vi "PCO_UserInterfaceSettings.vi"() -> (0 "PCO_UserInterfaceSettings":T2, 1 "PCO_UserInterfaceSettings_Raw":T1, 2 "Length":u16, 3 "Raw_Length":u16)   [LabVIEW 2020, in "SDK.lvlib" / "Structures.lvlib"]
doc: "Use this template to build a VI to use as a subVI."
uses:
  Structures.lvlib
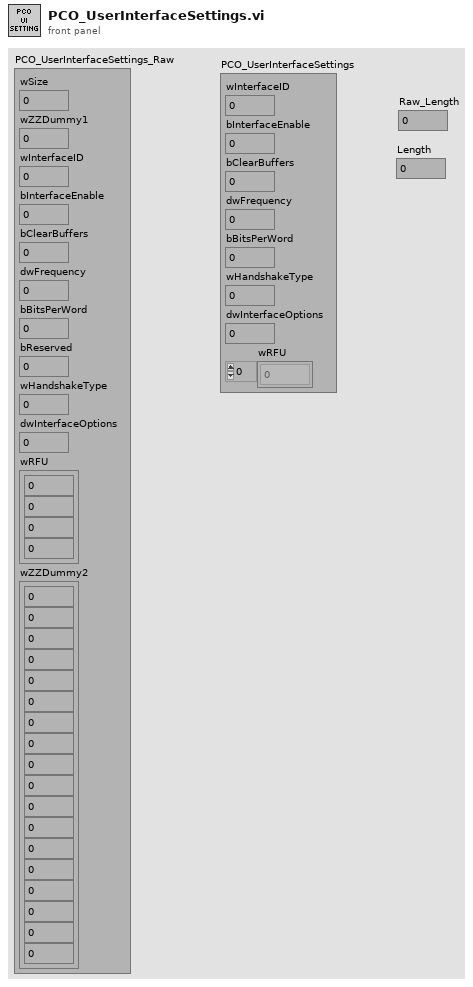
[diagram p1: front panel]
types:
  T1 = cluster{"wSize":u16, "wZZDummy1":u16, "wInterfaceID":u16, "bInterfaceEnable":u8, "bClearBuffers":u8, "dwFrequency":u32, "bBitsPerWord":u8, "bReserved":u8, "wHandshakeType":u16, "dwInterfaceOptions":u32, "wRFU":cluster{u16, u16, u16, u16}, "wZZDummy2":cluster{u16, u16, u16, u16, u16, u16, u16, u16, u16, u16, u16, u16, u16, u16, u16, u16, u16, u16}}
  T2 = cluster{"wInterfaceID":u16, "bInterfaceEnable":u8, "bClearBuffers":u8, "dwFrequency":u32, "bBitsPerWord":u8, "wHandshakeType":u16, "dwInterfaceOptions":u32, "wRFU":u16[]}
  T3 = cluster{u16, u16, u16, u16, u16, u16, u16, u16, u16, u16, u16, u16, u16, u16, u16, u16, u16, u16}
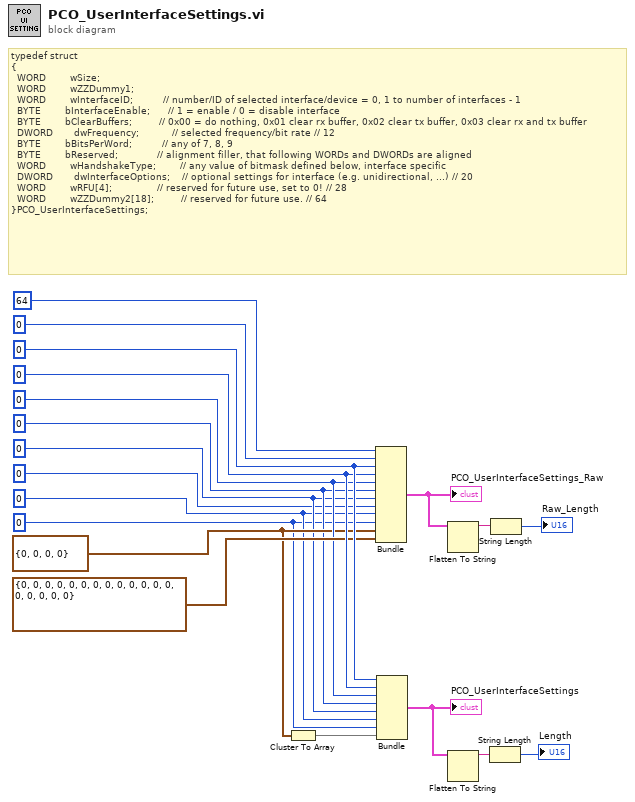
[diagram p0: block diagram]
diagram:
  w7 = cluster{u16, u16, u16, u16} {0, 0, 0, 0} ("wRFU")
  w2 = u32 0 ("dwInterfaceOptions")
  w3 = u16 0 ("wHandshakeType")
  w5 = u8 0 ("bBitsPerWord")
  w6 = u32 0 ("dwFrequency")
  w9 = u8 0 ("bClearBuffers")
  w12 = u8 0 ("bInterfaceEnable")
  w13 = u16 0 ("wInterfaceID")
  # "typedef struct\n{\n  WORD        wSize;\n  WORD        wZZDummy1;\n  WORD        wInterfaceID;          // number/ID of selected interface/device = 0, 1 to number of interfaces - 1\n  BYTE        bInterfaceEnable;      // 1 = enable / 0 = disable interface\n  BYTE        bClearBuffers;         // 0x00 = do nothing, 0x01 clear rx buffer, 0x02 clear tx buffer, 0x03 clear rx and tx buffer\n  DWORD       dwFrequency;           // selected frequency/bit rate // 12\n  BYTE        bBitsPerWord;          // any of 7, 8, 9\n  BYTE        bReserved;             // alignment filler, that following WORDs and DWORDs are aligned \n  WORD        wHandshakeType;        // any value of bitmask defined below, interface specific\n  DWORD       dwInterfaceOptions;    // optional settings for interface (e.g. unidirectional, ...) // 20\n  WORD        wRFU[4];               // reserved for future use, set to 0! // 28\n  WORD        wZZDummy2[18];         // reserved for future use. // 64\n}PCO_UserInterfaceSettings;"
  n1 = Cluster To Array(cluster=w7) -> (array=w1:u16[])
  n2 = Bundle("wSize"=u16 64, "wZZDummy1"=u16 0, "wInterfaceID"=w13, "bInterfaceEnable"=w12, "bClearBuffers"=w9, "dwFrequency"=w6, "bBitsPerWord"=w5, "bReserved"=u8 0, "wHandshakeType"=w3, "dwInterfaceOptions"=w2, "wRFU"=w7, "wZZDummy2"=T3 {0, 0, 0, 0, 0, 0, 0, 0, 0, 0, 0, 0, 0, 0, 0, 0, 0, 0}) -> (w14:T1)  [unwired: 1 in]
  "PCO_UserInterfaceSettings_Raw" <- w14
  n3 = Bundle("wInterfaceID"=w13, "bInterfaceEnable"=w12, "bClearBuffers"=w9, "dwFrequency"=w6, "bBitsPerWord"=w5, "wHandshakeType"=w3, "dwInterfaceOptions"=w2, "wRFU"=w1) -> (w8:T2)  [unwired: 1 in]
  "PCO_UserInterfaceSettings" <- w8
  n4 = Flatten To String(anything=w14) -> (data string=w18:string)  [unwired: 3 in, 2 out]
  n5 = Flatten To String(anything=w8) -> (data string=w19:string)  [unwired: 3 in, 2 out]
  n6 = String Length(string=w19) -> (length=→"Length":i32)
  n7 = String Length(string=w18) -> (length=→"Raw_Length":i32)
